vi "Get Socket DAQ Column Data.vi"(8 "error In":errorcluster, 9 "columns":string[](array[string])=["PhysicalChannel"], 10 "ChannelType":string="PWM_Input") -> (0 "error out":errorcluster, 2 "Data":string[][](array[string]))   [LabVIEW 2023, in "HardwareAbstractionLayer_LVOOP.lvlib" / "Teststand.lvclass"]
doc: "This VI Filter Physical Channel and Number Socket Running"
uses:
  Teststand.lvclass
  Database/Database.lvclass
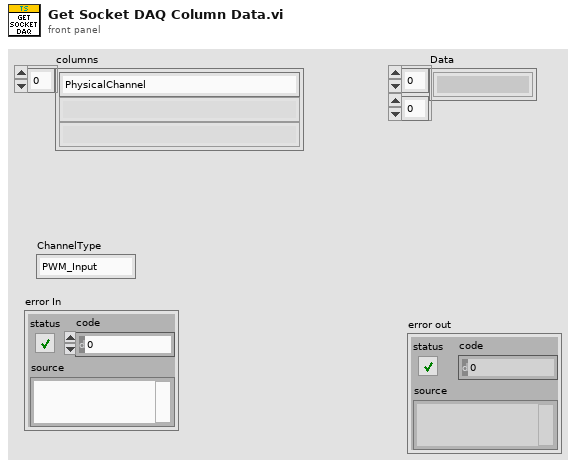
[diagram p1: front panel]
types:
  T1 = typedef "HardwareAbstractionLayer_LVOOP.lvlib/Teststand.lvclass/Teststand Status Control.ctl" = cluster{"Terminating or Aborting":bool, "Stop":bool, "Socket Count":i16, "Selected Sockets":i16[]}
  T2 = cluster{"table":string, "condition":string, "columns":string[]}
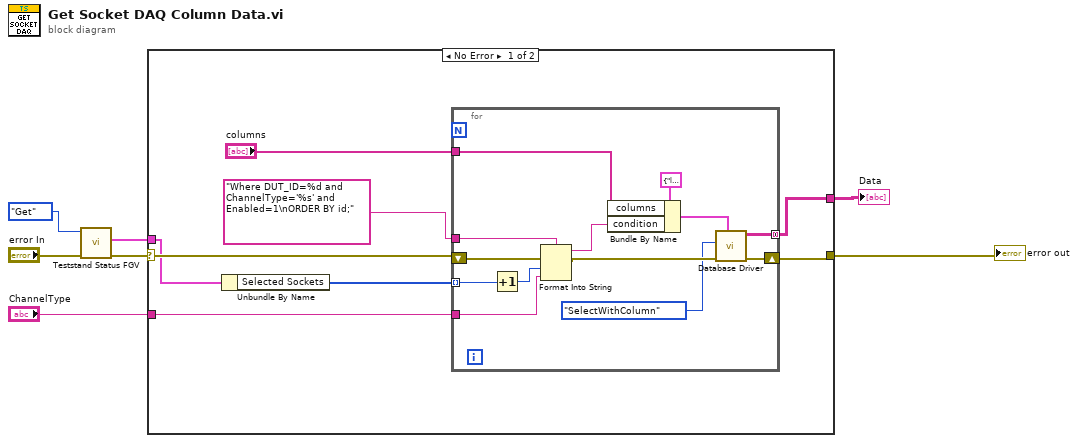
[diagram p0: block diagram]
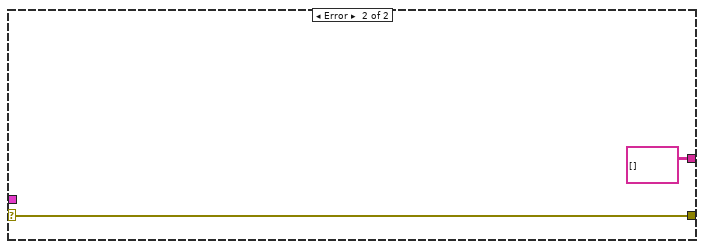
[diagram p2: hidden frame]
diagram:
  n1 = call "Teststand Status FGV.vi"("error in"="error In", "Option"=enum16{"Set", "Get"}."Get") -> ("error out"=w3:errorcluster, "Teststand Status Out"=w2:T1)  [unwired: 8 in]
  n2 = case shown="No Error" w3 {
    selector: w3 -> [w14 w30]
    tunnel: "ChannelType" -> [w13 _]
    tunnel: [w9 w30] -> w6
    tunnel: w2 -> [w12 _]
    tunnel: [w8 string[][] [] ("data")] -> w1
    frame No Error {
      n3 = Unbundle By Name(w12) -> ("Selected Sockets"=w11:i16[])
      n4 = for {
        tunnel: "Where DUT_ID=%d and ChannelType='%s' and Enabled=1\nORDER BY id;" -> [w28]
        shift-right: [w20] -> w9
        shift-left: w14 -> [w24]
        tunnel: [w19] -> w8 mode=concatenating
        tunnel: w13 -> [w23]
        tunnel: w11 -> [w17] mode=indexing
        tunnel: "columns" -> [w16]
        n5 = Increment(x=w17) -> (x+1=w27:i16)
        n6 = Format Into String(format string=w28, error in=w24, w27, w23) -> (resulting string=w25:string, error out=w21:errorcluster)  [unwired: 1 in]
        n7 = Bundle By Name(cluster=T2 {"table"="ltt.daq_configuration", "condition"="", "columns"=["PhysicalChannel"]} ("SQLTableData"), "columns"=w16, "condition"=w25) -> (w22:T2)
        n8 = call "Database Driver.vi"("SQLTableData"=w22, "error in"=w21, "Select"=enum16{"SelectWithQuery", "SelectWithColumn"}."SelectWithColumn") -> ("error out"=w20:errorcluster, "data"=w19:string[][])  [unwired: 5 in, 2 out]
      }
    }
    frame Error {
    }
  }
  "error out" <- w6
  "Data" <- w1
